vi "ServoCreate.vi"(8 "error in":errorcluster) -> (0 "error out":errorcluster, 3 "Device Out":i32)   [LabVIEW 2012]
uses:
  phidget21.dll
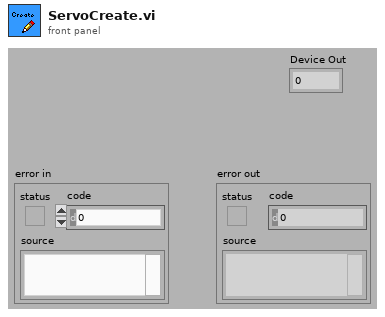
[diagram p1: front panel]
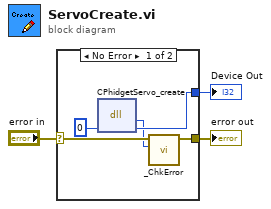
[diagram p0: block diagram]
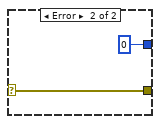
[diagram p2: hidden frame]
diagram:
  n1 = case shown="No Error" "error in" {
    selector: "error in" -> [w6 w10]
    tunnel: [w5 w10] -> w2
    tunnel: [w7 0 ("return type")] -> w1
    frame No Error {
      n2 = dll-call lib="phidget21.*" fn="CPhidgetServo_create"("phid"=0) -> (w4:i32, "phid"=w7:i32)  [unwired: 3 in, 2 out]
      n3 = call "_ChkError.vi"("Return Code"=w4, "error in (no error)"=w6) -> ("error out"=w5:errorcluster)  [unwired: 9 in]
    }
    frame Error {
    }
  }
  "error out" <- w2
  "Device Out" <- w1
